vi "WritePLC.vi"(5 "Ctrl Signals":T1, 7 "PLC IP address":string="192.168.1.52", 8 "Error In":errorcluster, 11 "PLCSignals In":T1) -> (0 "Error Out":errorcluster, 3 "PLCSignals Out":T1)   [LabVIEW 2018]
uses:
  Clusters/CtrlSignals.ctl
  <vilib>/ethernetip/ethernetip.llb/EthernetIP Tag Write BOOL.vi
  <vilib>/ethernetip/ethernetip.llb/EthernetIP Tag Write DINT.vi
  <vilib>/ethernetip/ethernetip.lvlib
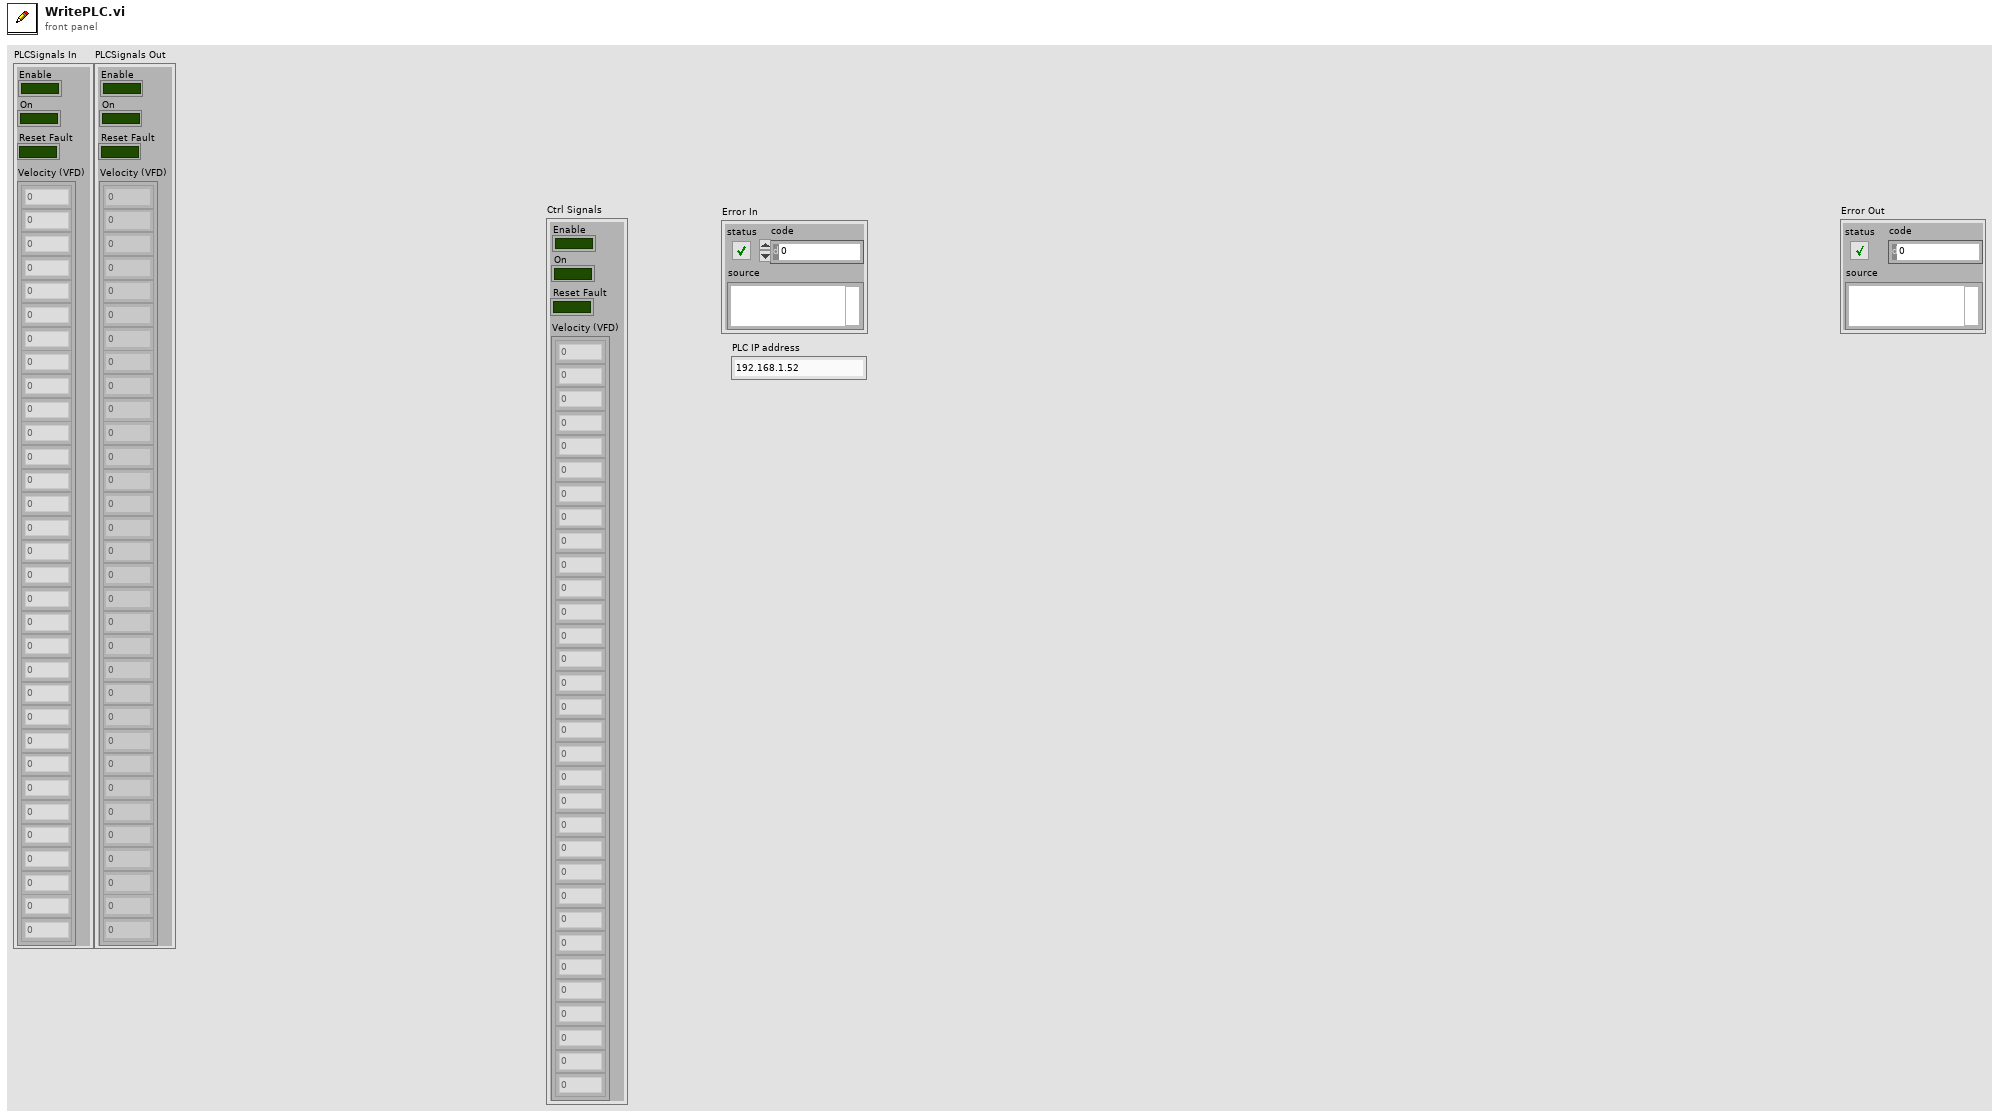
[diagram p1: front panel]
types:
  T1 = typedef "CtrlSignals.ctl" = cluster{"Enable":bool, "On":bool, "Reset Fault":bool, "Velocity (VFD)":i32[]}
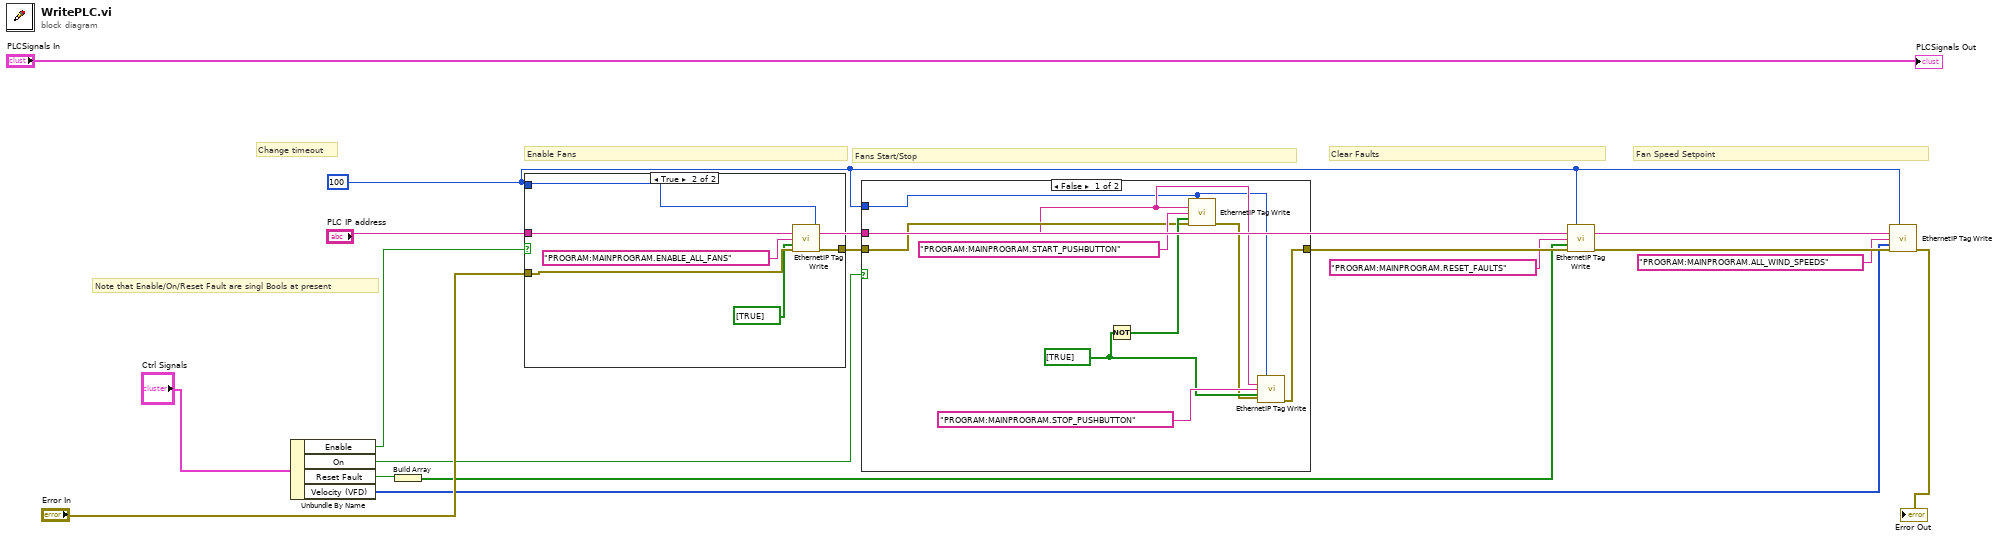
[diagram p0: block diagram]
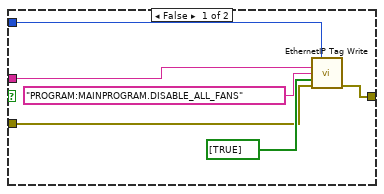
[diagram p2: hidden frame]
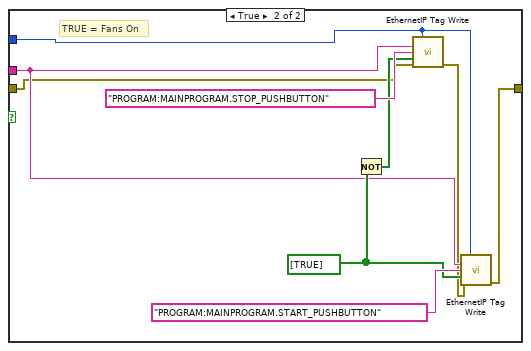
[diagram p3: hidden frame]
diagram:
  w9 = 100 ("Timeout (ms)")
  # "Fan Speed Setpoint"
  # "Clear Faults"
  # "Fans Start/Stop"
  # "Enable Fans"
  # "Note that Enable/On/Reset Fault are singl Bools at present"
  # "Change timeout"
  n1 = Unbundle By Name("Ctrl Signals") -> ("Enable"=w6:bool, "On"=w5:bool, "Reset Fault"=w10:bool, "Velocity (VFD)"=w3:i32[])
  n2 = Build Array(w10) -> (w4:bool[])
  n3 = case shown="True" w6 {
    tunnel: [w20 w27] -> w16
    tunnel: "PLC IP address" -> [w22 w26]
    tunnel: w9 -> [w21 w25]
    tunnel: "Error In" -> [w17 w24]
    frame False {
      n4 = call-poly <vilib>:"EthernetIP Tag Write.vi"("Timeout (ms)"=w21, "Network Path"=w22, "Tag Name"="PROGRAM:MAINPROGRAM.DISABLE_ALL_FANS", "Data"=bool[] [TRUE], "error in"=w17) -> ("error out"=w20:errorcluster)  [unwired: 9 in, 1 out]
    }
    frame True {
      n5 = call-poly <vilib>:"EthernetIP Tag Write.vi"("Timeout (ms)"=w25, "Network Path"=w26, "Tag Name"="PROGRAM:MAINPROGRAM.ENABLE_ALL_FANS", "Data"=bool[] [TRUE], "error in"=w24) -> ("error out"=w27:errorcluster)  [unwired: 9 in, 1 out]
    }
  }
  n6 = case shown="False" w5 {
    tunnel: w16 -> [w33 w40]
    tunnel: [w31 w38] -> w15
    tunnel: "PLC IP address" -> [w30 w41]
    tunnel: w9 -> [w29 w43]
    frame False {
      w35 = bool[] [TRUE] ("Data")
      n7 = Not(x=w35) -> (.not. x?=w34:bool[])
      n8 = call-poly <vilib>:"EthernetIP Tag Write.vi"("Timeout (ms)"=w29, "Network Path"=w30, "Tag Name"="PROGRAM:MAINPROGRAM.START_PUSHBUTTON", "Data"=w34, "error in"=w33) -> ("error out"=w32:errorcluster)  [unwired: 9 in, 1 out]
      n9 = call-poly <vilib>:"EthernetIP Tag Write.vi"("Timeout (ms)"=w29, "Network Path"=w30, "Tag Name"="PROGRAM:MAINPROGRAM.STOP_PUSHBUTTON", "Data"=w35, "error in"=w32) -> ("error out"=w31:errorcluster)  [unwired: 9 in, 1 out]
    }
    frame True {
      w44 = bool[] [TRUE] ("Data")
      # "TRUE = Fans On"
      n10 = Not(x=w44) -> (.not. x?=w42:bool[])
      n11 = call-poly <vilib>:"EthernetIP Tag Write.vi"("Timeout (ms)"=w43, "Network Path"=w41, "Tag Name"="PROGRAM:MAINPROGRAM.STOP_PUSHBUTTON", "Data"=w42, "error in"=w40) -> ("error out"=w39:errorcluster)  [unwired: 9 in, 1 out]
      n12 = call-poly <vilib>:"EthernetIP Tag Write.vi"("Timeout (ms)"=w43, "Network Path"=w41, "Tag Name"="PROGRAM:MAINPROGRAM.START_PUSHBUTTON", "Data"=w44, "error in"=w39) -> ("error out"=w38:errorcluster)  [unwired: 9 in, 1 out]
    }
  }
  n13 = call-poly <vilib>:"EthernetIP Tag Write.vi"("Timeout (ms)"=w9, "Network Path"="PLC IP address", "Tag Name"="PROGRAM:MAINPROGRAM.RESET_FAULTS", "Data"=w4, "error in"=w15) -> ("error out"=w13:errorcluster)  [unwired: 9 in, 1 out]
  n14 = call-poly <vilib>:"EthernetIP Tag Write.vi"("Timeout (ms)"=w9, "Network Path"="PLC IP address", "Tag Name"="PROGRAM:MAINPROGRAM.ALL_WIND_SPEEDS", "Data"=w3, "error in"=w13) -> ("error out"=→"Error Out":errorcluster)  [unwired: 9 in, 1 out]
  "PLCSignals Out" <- "PLCSignals In"
